vi "XLP80_Action_InitListboxes.vi"(8 "err in":errorcluster) -> (0 "err out":errorcluster)   [LabVIEW 2021]
uses:
  XLP80_State_V001.llb/XLP80_State_TDefEnumGlobalState.ctl
  <vilib>/Utility/miscctls.llb/LVRowAndColumnUnsignedTypeDef.ctl
  XLP80_Globals/Globals_Settings_XLP80.vi
  XLP80_Globals/XLP80_Globals_Referenzen.vi
  XLP80_Globals/XLP80_CAN_Globals.vi
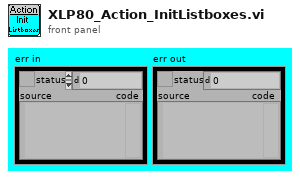
[diagram p1: front panel]
types:
  T1 = typedef "XLP80_State_TDefEnumGlobalState.ctl" = enum16{"HV & Software", "Basis Funktion", "Power Management", "Operational Mode", "Shutdown", "Alarm"}
  T2 = cluster{"Signal Name":string[], "Description":string[], "Unit":string[], "Min":dbl[], "Max":dbl[], "HV & Software":bool[], "Basis Funktion":bool[], "Power Management":bool[], "OperationMode":bool[], "Shutdown":bool[], "Alarm":bool[], "LogEnable":bool[]}
  T3 = typedef "LVRowAndColumnUnsignedTypeDef.ctl" = cluster{"Row":u32, "Column":u32}
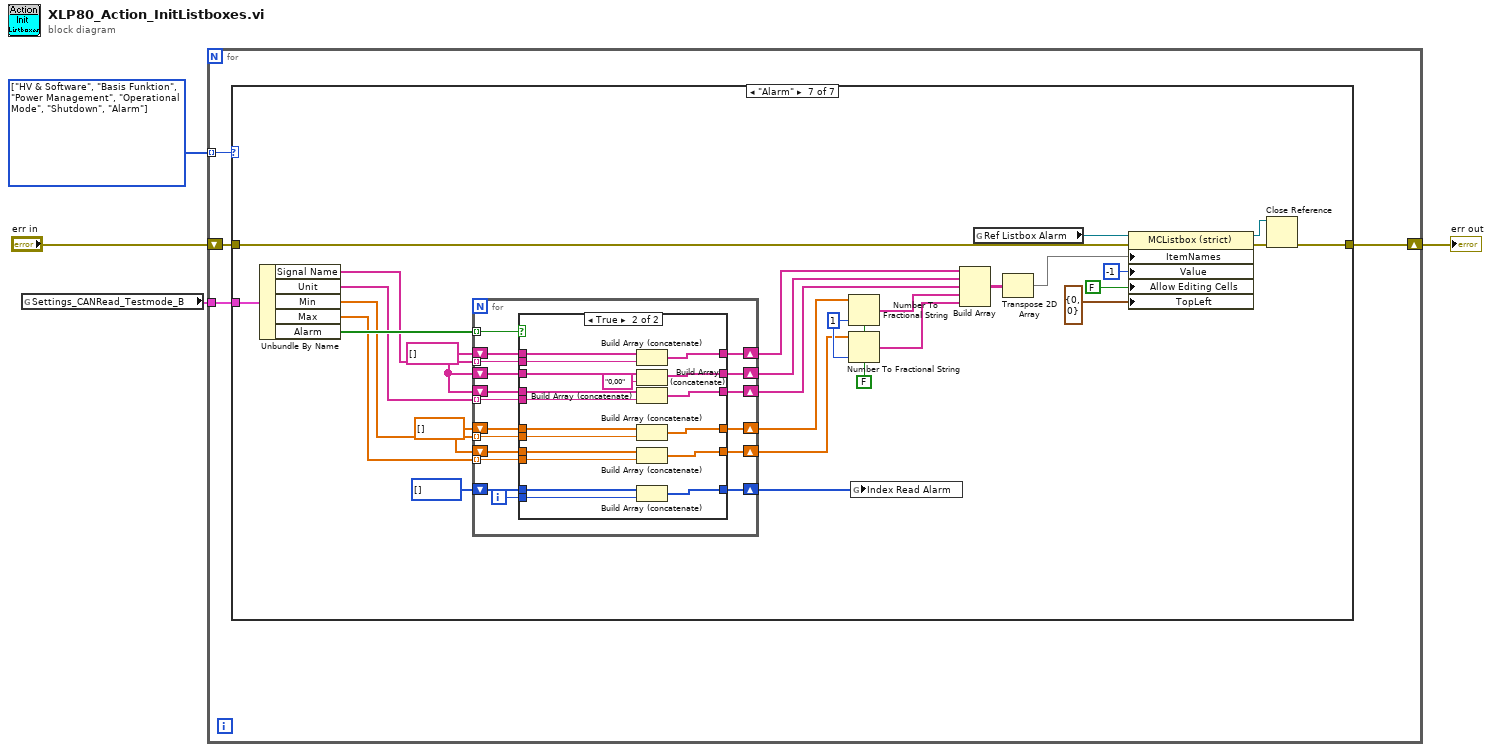
[diagram p0: block diagram]
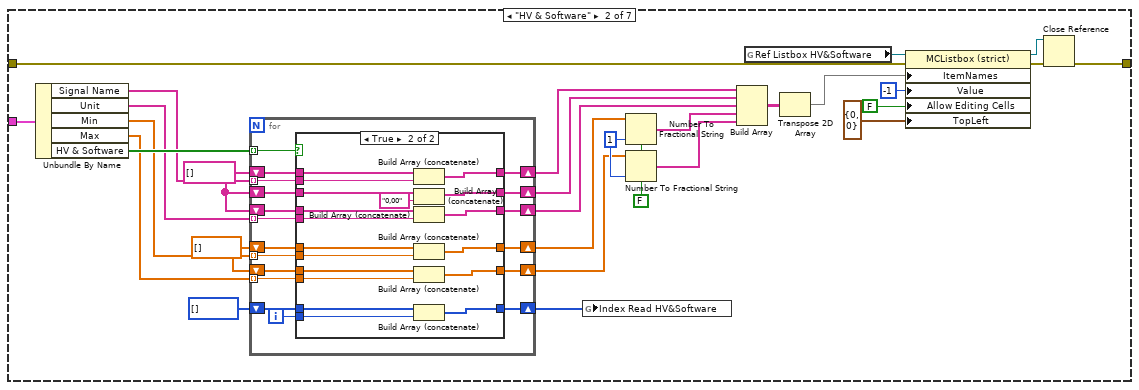
[diagram p3: hidden frame]
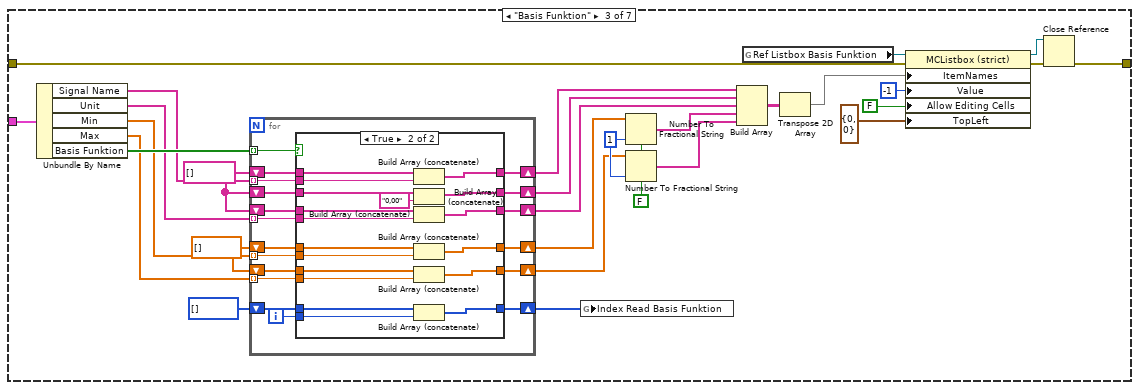
[diagram p5: hidden frame]
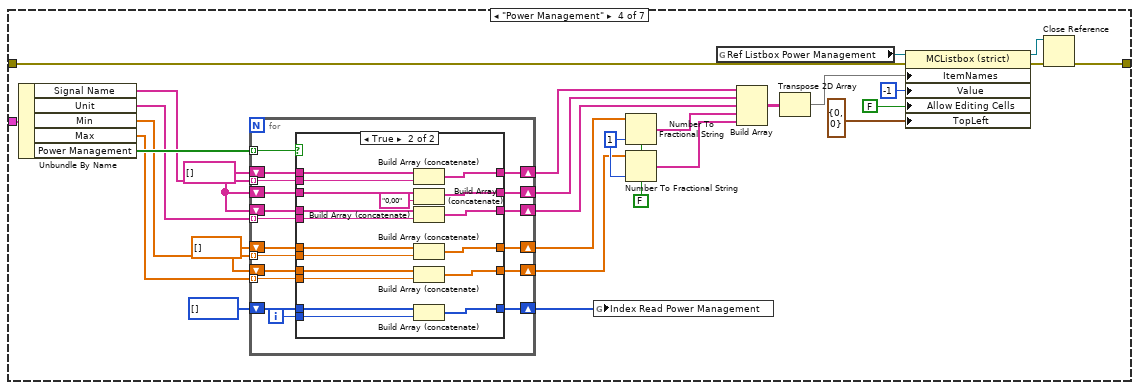
[diagram p7: hidden frame]
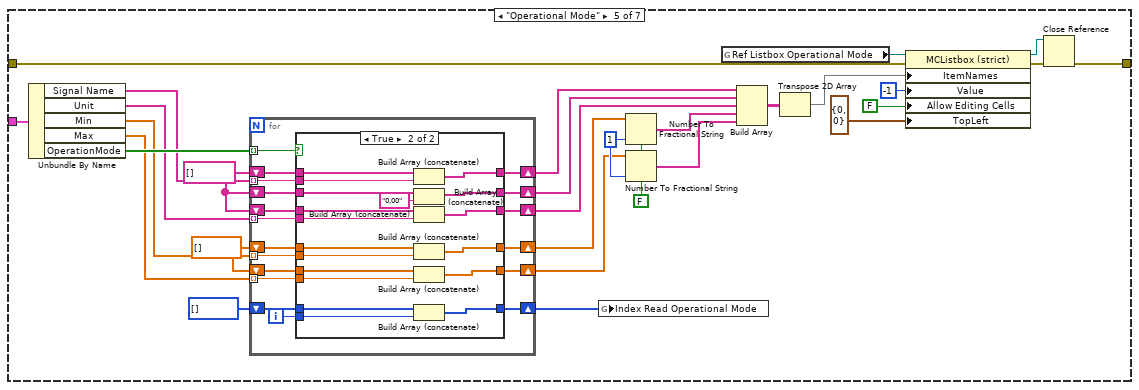
[diagram p9: hidden frame]
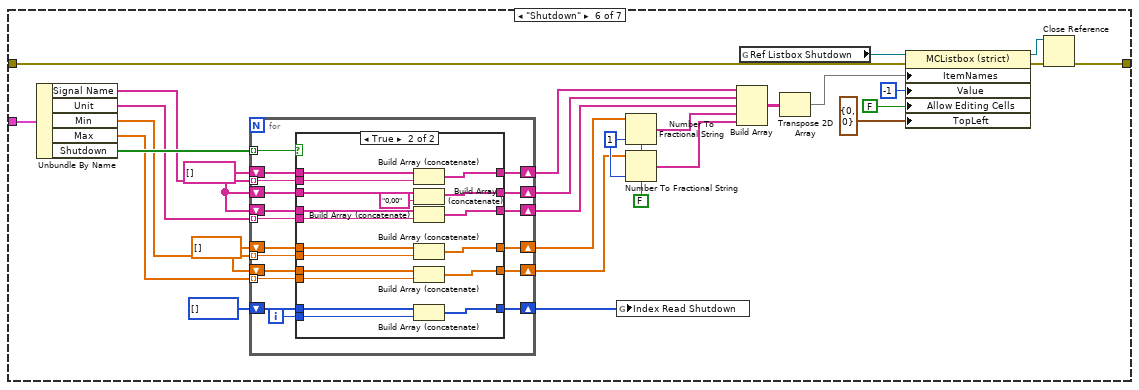
[diagram p11: hidden frame]
diagram:
  w1 = T1[] [enum."HV & Software", enum."Basis Funktion", enum."Power Management", enum."Operational Mode", enum."Shutdown", enum."Alarm"] items=["HV & Software", "Basis Funktion", "Power Management", "Operational Mode", "Shutdown", "Alarm"]
  n1 = global read "Globals_Settings_XLP80.vi" "Settings_CANRead_Testmode_B"() -> (w4:T2)
  n2 = for {
    tunnel: w4 -> [w8]
    shift-right: [w7] -> w3
    shift-left: "err in" -> [w6]
    tunnel: w1 -> [w5] mode=indexing
    n3 = case shown="\"Alarm\"" w5 {
      tunnel: w8 -> [_ w38 w109 w180 w251 w322 w393]
      tunnel: [w9 w26 w97 w168 w239 w310 w381] -> w7
      tunnel: w6 -> [w9 w25 w96 w167 w238 w309 w380]
      frame Default {
      }
      frame "HV & Software" {
        w18 = dbl[] [] ("Max")
        w21 = string[] [] ("Signal Name")
        w30 = i16 1 ("precision (6)")
        w31 = FALSE ("use system decimal point (T)")
        n4 = Unbundle By Name(w38) -> ("Signal Name"=w22:string[], "Unit"=w20:string[], "Min"=w19:dbl[], "Max"=w17:dbl[], "HV & Software"=w24:bool[])
        n5 = for {
          tunnel: w24 -> [w56] mode=indexing
          shift-right: [w53] -> w16
          shift-left: w21 -> [w55]
          shift-right: [w39] -> w11
          shift-left: i32[] [] -> [w44]
          tunnel: w22 -> [w54] mode=indexing
          shift-right: [w51] -> w15
          shift-left: w21 -> [w52]
          shift-right: [w48] -> w14
          shift-left: w21 -> [w50]
          tunnel: w20 -> [w49] mode=indexing
          shift-right: [w45] -> w13
          shift-left: w18 -> [w47]
          tunnel: w19 -> [w46] mode=indexing
          shift-right: [w40] -> w12
          shift-left: w18 -> [w42]
          tunnel: w17 -> [w41] mode=indexing
          i -> [w43]
          n6 = case shown="True" w56 {
            tunnel: w55 -> [w62 w80]
            tunnel: w54 -> [_ w79]
            tunnel: [w62 w78] -> w53
            tunnel: w52 -> [w61 w77]
            tunnel: [w61 w76] -> w51
            tunnel: w50 -> [w60 w74]
            tunnel: w49 -> [_ w73]
            tunnel: [w60 w72] -> w48
            tunnel: w47 -> [w59 w71]
            tunnel: w46 -> [_ w70]
            tunnel: [w59 w69] -> w45
            tunnel: w44 -> [w57 w68]
            tunnel: w43 -> [_ w67]
            tunnel: w42 -> [w58 w66]
            tunnel: w41 -> [_ w65]
            tunnel: [w58 w64] -> w40
            tunnel: [w57 w63] -> w39
            frame False {
            }
            frame True {
              n7 = Build Array (concatenate)(w80, w79) -> (w78:string[])
              n8 = Build Array (concatenate)(w77, "0,00") -> (w76:string[])
              n9 = Build Array (concatenate)(w74, w73) -> (w72:string[])
              n10 = Build Array (concatenate)(w71, w70) -> (w69:dbl[])
              n11 = Build Array (concatenate)(w66, w65) -> (w64:dbl[])
              n12 = Build Array (concatenate)(w68, w67) -> (w63:i32[])
            }
          }
        }
        n13 = global write "XLP80_CAN_Globals.vi" "Index Read HV&Software"(w11) -> ()
        n14 = Number To Fractional String(use system decimal point (T)=w31, number=w13, precision (6)=w30) -> (F-format string=w37:string[])  [unwired: 1 in]
        n15 = Number To Fractional String(use system decimal point (T)=w31, number=w12, precision (6)=w30) -> (F-format string=w36:string[])  [unwired: 1 in]
        n16 = Build Array(w16, w15, w14, w37, w36) -> (w35:string[][])
        n17 = global read "XLP80_Globals_Referenzen.vi" "Ref Listbox HV&Software"() -> (w27:refnum<vi>)
        n18 = Transpose 2D Array(2D array=w35) -> (transposed array=w34:string[][])
        n19 = property class="MCListbox (strict)"(reference=w27, error in=w25, "ItemNames"=w34, "Value"=-1, "Allow Editing Cells"=FALSE, "TopLeft"=T3 {"Row"=0, "Column"=0} ("Top Left Visible Cell")) -> (reference out=w32:refnum<vi>, error out=w33:errorcluster)
        n20 = Close Reference(reference=w32, error in (no error)=w33) -> (error out=w26:errorcluster)
      }
      frame "Basis Funktion" {
        w89 = dbl[] [] ("Max")
        w92 = string[] [] ("Signal Name")
        w101 = i16 1 ("precision (6)")
        w102 = FALSE ("use system decimal point (T)")
        n21 = Unbundle By Name(w109) -> ("Signal Name"=w93:string[], "Unit"=w91:string[], "Min"=w90:dbl[], "Max"=w88:dbl[], "Basis Funktion"=w95:bool[])
        n22 = for {
          tunnel: w95 -> [w127] mode=indexing
          shift-right: [w124] -> w87
          shift-left: w92 -> [w126]
          shift-right: [w110] -> w82
          shift-left: i32[] [] -> [w115]
          tunnel: w93 -> [w125] mode=indexing
          shift-right: [w122] -> w86
          shift-left: w92 -> [w123]
          shift-right: [w119] -> w85
          shift-left: w92 -> [w121]
          tunnel: w91 -> [w120] mode=indexing
          shift-right: [w116] -> w84
          shift-left: w89 -> [w118]
          tunnel: w90 -> [w117] mode=indexing
          shift-right: [w111] -> w83
          shift-left: w89 -> [w113]
          tunnel: w88 -> [w112] mode=indexing
          i -> [w114]
          n23 = case shown="True" w127 {
            tunnel: w126 -> [w133 w151]
            tunnel: w125 -> [_ w150]
            tunnel: [w133 w149] -> w124
            tunnel: w123 -> [w132 w148]
            tunnel: [w132 w147] -> w122
            tunnel: w121 -> [w131 w145]
            tunnel: w120 -> [_ w144]
            tunnel: [w131 w143] -> w119
            tunnel: w118 -> [w130 w142]
            tunnel: w117 -> [_ w141]
            tunnel: [w130 w140] -> w116
            tunnel: w115 -> [w128 w139]
            tunnel: w114 -> [_ w138]
            tunnel: w113 -> [w129 w137]
            tunnel: w112 -> [_ w136]
            tunnel: [w129 w135] -> w111
            tunnel: [w128 w134] -> w110
            frame False {
            }
            frame True {
              n24 = Build Array (concatenate)(w151, w150) -> (w149:string[])
              n25 = Build Array (concatenate)(w148, "0,00") -> (w147:string[])
              n26 = Build Array (concatenate)(w145, w144) -> (w143:string[])
              n27 = Build Array (concatenate)(w142, w141) -> (w140:dbl[])
              n28 = Build Array (concatenate)(w137, w136) -> (w135:dbl[])
              n29 = Build Array (concatenate)(w139, w138) -> (w134:i32[])
            }
          }
        }
        n30 = global write "XLP80_CAN_Globals.vi" "Index Read Basis Funktion"(w82) -> ()
        n31 = Number To Fractional String(use system decimal point (T)=w102, number=w84, precision (6)=w101) -> (F-format string=w108:string[])  [unwired: 1 in]
        n32 = Number To Fractional String(use system decimal point (T)=w102, number=w83, precision (6)=w101) -> (F-format string=w107:string[])  [unwired: 1 in]
        n33 = Build Array(w87, w86, w85, w108, w107) -> (w106:string[][])
        n34 = global read "XLP80_Globals_Referenzen.vi" "Ref Listbox Basis Funktion"() -> (w98:refnum<vi>)
        n35 = Transpose 2D Array(2D array=w106) -> (transposed array=w105:string[][])
        n36 = property class="MCListbox (strict)"(reference=w98, error in=w96, "ItemNames"=w105, "Value"=-1, "Allow Editing Cells"=FALSE, "TopLeft"=T3 {"Row"=0, "Column"=0} ("Top Left Visible Cell")) -> (reference out=w103:refnum<vi>, error out=w104:errorcluster)
        n37 = Close Reference(reference=w103, error in (no error)=w104) -> (error out=w97:errorcluster)
      }
      frame "Power Management" {
        w160 = dbl[] [] ("Max")
        w163 = string[] [] ("Signal Name")
        w172 = i16 1 ("precision (6)")
        w173 = FALSE ("use system decimal point (T)")
        n38 = Unbundle By Name(w180) -> ("Signal Name"=w164:string[], "Unit"=w162:string[], "Min"=w161:dbl[], "Max"=w159:dbl[], "Power Management"=w166:bool[])
        n39 = for {
          tunnel: w166 -> [w198] mode=indexing
          shift-right: [w195] -> w158
          shift-left: w163 -> [w197]
          shift-right: [w181] -> w153
          shift-left: i32[] [] -> [w186]
          tunnel: w164 -> [w196] mode=indexing
          shift-right: [w193] -> w157
          shift-left: w163 -> [w194]
          shift-right: [w190] -> w156
          shift-left: w163 -> [w192]
          tunnel: w162 -> [w191] mode=indexing
          shift-right: [w187] -> w155
          shift-left: w160 -> [w189]
          tunnel: w161 -> [w188] mode=indexing
          shift-right: [w182] -> w154
          shift-left: w160 -> [w184]
          tunnel: w159 -> [w183] mode=indexing
          i -> [w185]
          n40 = case shown="True" w198 {
            tunnel: w197 -> [w204 w222]
            tunnel: w196 -> [_ w221]
            tunnel: [w204 w220] -> w195
            tunnel: w194 -> [w203 w219]
            tunnel: [w203 w218] -> w193
            tunnel: w192 -> [w202 w216]
            tunnel: w191 -> [_ w215]
            tunnel: [w202 w214] -> w190
            tunnel: w189 -> [w201 w213]
            tunnel: w188 -> [_ w212]
            tunnel: [w201 w211] -> w187
            tunnel: w186 -> [w199 w210]
            tunnel: w185 -> [_ w209]
            tunnel: w184 -> [w200 w208]
            tunnel: w183 -> [_ w207]
            tunnel: [w200 w206] -> w182
            tunnel: [w199 w205] -> w181
            frame False {
            }
            frame True {
              n41 = Build Array (concatenate)(w222, w221) -> (w220:string[])
              n42 = Build Array (concatenate)(w219, "0,00") -> (w218:string[])
              n43 = Build Array (concatenate)(w216, w215) -> (w214:string[])
              n44 = Build Array (concatenate)(w213, w212) -> (w211:dbl[])
              n45 = Build Array (concatenate)(w208, w207) -> (w206:dbl[])
              n46 = Build Array (concatenate)(w210, w209) -> (w205:i32[])
            }
          }
        }
        n47 = global write "XLP80_CAN_Globals.vi" "Index Read Power Management"(w153) -> ()
        n48 = Number To Fractional String(use system decimal point (T)=w173, number=w155, precision (6)=w172) -> (F-format string=w179:string[])  [unwired: 1 in]
        n49 = Number To Fractional String(use system decimal point (T)=w173, number=w154, precision (6)=w172) -> (F-format string=w178:string[])  [unwired: 1 in]
        n50 = global read "XLP80_Globals_Referenzen.vi" "Ref Listbox Power Management"() -> (w169:refnum<vi>)
        n51 = Build Array(w158, w157, w156, w179, w178) -> (w177:string[][])
        n52 = Transpose 2D Array(2D array=w177) -> (transposed array=w176:string[][])
        n53 = property class="MCListbox (strict)"(reference=w169, error in=w167, "ItemNames"=w176, "Value"=-1, "Allow Editing Cells"=FALSE, "TopLeft"=T3 {"Row"=0, "Column"=0} ("Top Left Visible Cell")) -> (reference out=w174:refnum<vi>, error out=w175:errorcluster)
        n54 = Close Reference(reference=w174, error in (no error)=w175) -> (error out=w168:errorcluster)
      }
      frame "Operational Mode" {
        w231 = dbl[] [] ("Max")
        w234 = string[] [] ("Signal Name")
        w243 = i16 1 ("precision (6)")
        w244 = FALSE ("use system decimal point (T)")
        n55 = Unbundle By Name(w251) -> ("Signal Name"=w235:string[], "Unit"=w233:string[], "Min"=w232:dbl[], "Max"=w230:dbl[], "OperationMode"=w237:bool[])
        n56 = for {
          tunnel: w237 -> [w269] mode=indexing
          shift-right: [w266] -> w229
          shift-left: w234 -> [w268]
          shift-right: [w252] -> w224
          shift-left: i32[] [] -> [w257]
          tunnel: w235 -> [w267] mode=indexing
          shift-right: [w264] -> w228
          shift-left: w234 -> [w265]
          shift-right: [w261] -> w227
          shift-left: w234 -> [w263]
          tunnel: w233 -> [w262] mode=indexing
          shift-right: [w258] -> w226
          shift-left: w231 -> [w260]
          tunnel: w232 -> [w259] mode=indexing
          shift-right: [w253] -> w225
          shift-left: w231 -> [w255]
          tunnel: w230 -> [w254] mode=indexing
          i -> [w256]
          n57 = case shown="True" w269 {
            tunnel: w268 -> [w275 w293]
            tunnel: w267 -> [_ w292]
            tunnel: [w275 w291] -> w266
            tunnel: w265 -> [w274 w290]
            tunnel: [w274 w289] -> w264
            tunnel: w263 -> [w273 w287]
            tunnel: w262 -> [_ w286]
            tunnel: [w273 w285] -> w261
            tunnel: w260 -> [w272 w284]
            tunnel: w259 -> [_ w283]
            tunnel: [w272 w282] -> w258
            tunnel: w257 -> [w270 w281]
            tunnel: w256 -> [_ w280]
            tunnel: w255 -> [w271 w279]
            tunnel: w254 -> [_ w278]
            tunnel: [w271 w277] -> w253
            tunnel: [w270 w276] -> w252
            frame False {
            }
            frame True {
              n58 = Build Array (concatenate)(w293, w292) -> (w291:string[])
              n59 = Build Array (concatenate)(w290, "0,00") -> (w289:string[])
              n60 = Build Array (concatenate)(w287, w286) -> (w285:string[])
              n61 = Build Array (concatenate)(w284, w283) -> (w282:dbl[])
              n62 = Build Array (concatenate)(w279, w278) -> (w277:dbl[])
              n63 = Build Array (concatenate)(w281, w280) -> (w276:i32[])
            }
          }
        }
        n64 = global write "XLP80_CAN_Globals.vi" "Index Read Operational Mode"(w224) -> ()
        n65 = Number To Fractional String(use system decimal point (T)=w244, number=w226, precision (6)=w243) -> (F-format string=w250:string[])  [unwired: 1 in]
        n66 = Number To Fractional String(use system decimal point (T)=w244, number=w225, precision (6)=w243) -> (F-format string=w249:string[])  [unwired: 1 in]
        n67 = global read "XLP80_Globals_Referenzen.vi" "Ref Listbox Operational Mode"() -> (w240:refnum<vi>)
        n68 = Build Array(w229, w228, w227, w250, w249) -> (w248:string[][])
        n69 = Transpose 2D Array(2D array=w248) -> (transposed array=w247:string[][])
        n70 = property class="MCListbox (strict)"(reference=w240, error in=w238, "ItemNames"=w247, "Value"=-1, "Allow Editing Cells"=FALSE, "TopLeft"=T3 {"Row"=0, "Column"=0} ("Top Left Visible Cell")) -> (reference out=w245:refnum<vi>, error out=w246:errorcluster)
        n71 = Close Reference(reference=w245, error in (no error)=w246) -> (error out=w239:errorcluster)
      }
      frame "Shutdown" {
        w302 = dbl[] [] ("Max")
        w305 = string[] [] ("Signal Name")
        w314 = i16 1 ("precision (6)")
        w315 = FALSE ("use system decimal point (T)")
        n72 = Unbundle By Name(w322) -> ("Signal Name"=w306:string[], "Unit"=w304:string[], "Min"=w303:dbl[], "Max"=w301:dbl[], "Shutdown"=w308:bool[])
        n73 = for {
          tunnel: w308 -> [w340] mode=indexing
          shift-right: [w337] -> w300
          shift-left: w305 -> [w339]
          shift-right: [w323] -> w295
          shift-left: i32[] [] -> [w328]
          tunnel: w306 -> [w338] mode=indexing
          shift-right: [w335] -> w299
          shift-left: w305 -> [w336]
          shift-right: [w332] -> w298
          shift-left: w305 -> [w334]
          tunnel: w304 -> [w333] mode=indexing
          shift-right: [w329] -> w297
          shift-left: w302 -> [w331]
          tunnel: w303 -> [w330] mode=indexing
          shift-right: [w324] -> w296
          shift-left: w302 -> [w326]
          tunnel: w301 -> [w325] mode=indexing
          i -> [w327]
          n74 = case shown="True" w340 {
            tunnel: w339 -> [w346 w364]
            tunnel: w338 -> [_ w363]
            tunnel: [w346 w362] -> w337
            tunnel: w336 -> [w345 w361]
            tunnel: [w345 w360] -> w335
            tunnel: w334 -> [w344 w358]
            tunnel: w333 -> [_ w357]
            tunnel: [w344 w356] -> w332
            tunnel: w331 -> [w343 w355]
            tunnel: w330 -> [_ w354]
            tunnel: [w343 w353] -> w329
            tunnel: w328 -> [w341 w352]
            tunnel: w327 -> [_ w351]
            tunnel: w326 -> [w342 w350]
            tunnel: w325 -> [_ w349]
            tunnel: [w342 w348] -> w324
            tunnel: [w341 w347] -> w323
            frame False {
            }
            frame True {
              n75 = Build Array (concatenate)(w364, w363) -> (w362:string[])
              n76 = Build Array (concatenate)(w361, "0,00") -> (w360:string[])
              n77 = Build Array (concatenate)(w358, w357) -> (w356:string[])
              n78 = Build Array (concatenate)(w355, w354) -> (w353:dbl[])
              n79 = Build Array (concatenate)(w350, w349) -> (w348:dbl[])
              n80 = Build Array (concatenate)(w352, w351) -> (w347:i32[])
            }
          }
        }
        n81 = global write "XLP80_CAN_Globals.vi" "Index Read Shutdown"(w295) -> ()
        n82 = Number To Fractional String(use system decimal point (T)=w315, number=w297, precision (6)=w314) -> (F-format string=w321:string[])  [unwired: 1 in]
        n83 = Number To Fractional String(use system decimal point (T)=w315, number=w296, precision (6)=w314) -> (F-format string=w320:string[])  [unwired: 1 in]
        n84 = Build Array(w300, w299, w298, w321, w320) -> (w319:string[][])
        n85 = global read "XLP80_Globals_Referenzen.vi" "Ref Listbox Shutdown"() -> (w311:refnum<vi>)
        n86 = Transpose 2D Array(2D array=w319) -> (transposed array=w318:string[][])
        n87 = property class="MCListbox (strict)"(reference=w311, error in=w309, "ItemNames"=w318, "Value"=-1, "Allow Editing Cells"=FALSE, "TopLeft"=T3 {"Row"=0, "Column"=0} ("Top Left Visible Cell")) -> (reference out=w316:refnum<vi>, error out=w317:errorcluster)
        n88 = Close Reference(reference=w316, error in (no error)=w317) -> (error out=w310:errorcluster)
      }
      frame "Alarm" {
        w373 = dbl[] [] ("Max")
        w376 = string[] [] ("Signal Name")
        w385 = i16 1 ("precision (6)")
        w386 = FALSE ("use system decimal point (T)")
        n89 = Unbundle By Name(w393) -> ("Signal Name"=w377:string[], "Unit"=w375:string[], "Min"=w374:dbl[], "Max"=w372:dbl[], "Alarm"=w379:bool[])
        n90 = for {
          tunnel: w379 -> [w411] mode=indexing
          shift-right: [w408] -> w371
          shift-left: w376 -> [w410]
          shift-right: [w394] -> w366
          shift-left: i32[] [] -> [w399]
          tunnel: w377 -> [w409] mode=indexing
          shift-right: [w406] -> w370
          shift-left: w376 -> [w407]
          shift-right: [w403] -> w369
          shift-left: w376 -> [w405]
          tunnel: w375 -> [w404] mode=indexing
          shift-right: [w400] -> w368
          shift-left: w373 -> [w402]
          tunnel: w374 -> [w401] mode=indexing
          shift-right: [w395] -> w367
          shift-left: w373 -> [w397]
          tunnel: w372 -> [w396] mode=indexing
          i -> [w398]
          n91 = case shown="True" w411 {
            tunnel: w410 -> [w417 w435]
            tunnel: w409 -> [_ w434]
            tunnel: [w417 w433] -> w408
            tunnel: w407 -> [w416 w432]
            tunnel: [w416 w431] -> w406
            tunnel: w405 -> [w415 w429]
            tunnel: w404 -> [_ w428]
            tunnel: [w415 w427] -> w403
            tunnel: w402 -> [w414 w426]
            tunnel: w401 -> [_ w425]
            tunnel: [w414 w424] -> w400
            tunnel: w399 -> [w412 w423]
            tunnel: w398 -> [_ w422]
            tunnel: w397 -> [w413 w421]
            tunnel: w396 -> [_ w420]
            tunnel: [w413 w419] -> w395
            tunnel: [w412 w418] -> w394
            frame False {
            }
            frame True {
              n92 = Build Array (concatenate)(w435, w434) -> (w433:string[])
              n93 = Build Array (concatenate)(w432, "0,00") -> (w431:string[])
              n94 = Build Array (concatenate)(w429, w428) -> (w427:string[])
              n95 = Build Array (concatenate)(w426, w425) -> (w424:dbl[])
              n96 = Build Array (concatenate)(w421, w420) -> (w419:dbl[])
              n97 = Build Array (concatenate)(w423, w422) -> (w418:i32[])
            }
          }
        }
        n98 = Number To Fractional String(use system decimal point (T)=w386, number=w368, precision (6)=w385) -> (F-format string=w392:string[])  [unwired: 1 in]
        n99 = Number To Fractional String(use system decimal point (T)=w386, number=w367, precision (6)=w385) -> (F-format string=w391:string[])  [unwired: 1 in]
        n100 = global write "XLP80_CAN_Globals.vi" "Index Read Alarm"(w366) -> ()
        n101 = Build Array(w371, w370, w369, w392, w391) -> (w390:string[][])
        n102 = global read "XLP80_Globals_Referenzen.vi" "Ref Listbox Alarm"() -> (w382:refnum<vi>)
        n103 = Transpose 2D Array(2D array=w390) -> (transposed array=w389:string[][])
        n104 = property class="MCListbox (strict)"(reference=w382, error in=w380, "ItemNames"=w389, "Value"=-1, "Allow Editing Cells"=FALSE, "TopLeft"=T3 {"Row"=0, "Column"=0} ("Top Left Visible Cell")) -> (reference out=w387:refnum<vi>, error out=w388:errorcluster)
        n105 = Close Reference(reference=w387, error in (no error)=w388) -> (error out=w381:errorcluster)
      }
    }
  }
  "err out" <- w3
